vi "SpectrumAnalyzer.vi"() -> ()   [LabVIEW 2024]
uses:
  <vilib>/express/express analysis/Spectral/Block/exnSpectralBlock spectral measurements RMS poly.vi
  <vilib>/express/express analysis/Spectral/Block/exnSpectralBlock spectral measurements RMS WFM.vi
  <vilib>/express/express analysis/Spectral/XNode/ExpressSpectralMeasurementsBlockNode.xnode
  <vilib>/express/express analysis/Spectral/Block/exnSpectralBlock spectral measurements RMS DDT.vi
  <vilib>/Waveform/WDTOps.llb/WDT Waveform to XY Pairs DBL.vi
panel:
  out "Mic Wave 2":dynamicdata(graph) caption="Sine"
  out "mic+waves FFT":cluster{"f0":dbl, "df":dbl, "magnitude":dbl[]}(graph)
  out "Mic and waves SUM":waveform(dbl)(graph)
  in  "stop 2":bool
  in  "Simulate Waves Button":bool
  in  "Play Sound Button":bool
  out "Square Wave":dbl[](graph)
  out "Sine Wave":dbl[](graph)
  in  "Sin Coeffs":cluster{"freq":dbl, "Amp":dbl, "Phase":dbl}={"freq"=100.0, "Amp"=10.0, "Phase"=0.0}
  in  "Square Coeffs":cluster{"freq":dbl, "Amp":dbl, "Phase":dbl}={"freq"=100.0, "Amp"=10.0, "Phase"=0.0}
  in  "Sample Rate":dbl=44100.0
  in  "Duration":dbl=3.0
  in  "Signal Toggles":cluster{"Mic":bool, "Sin":bool, "Squ":bool}={"Mic"=TRUE, "Sin"=TRUE, "Squ"=TRUE}
  in  "Record Button":bool
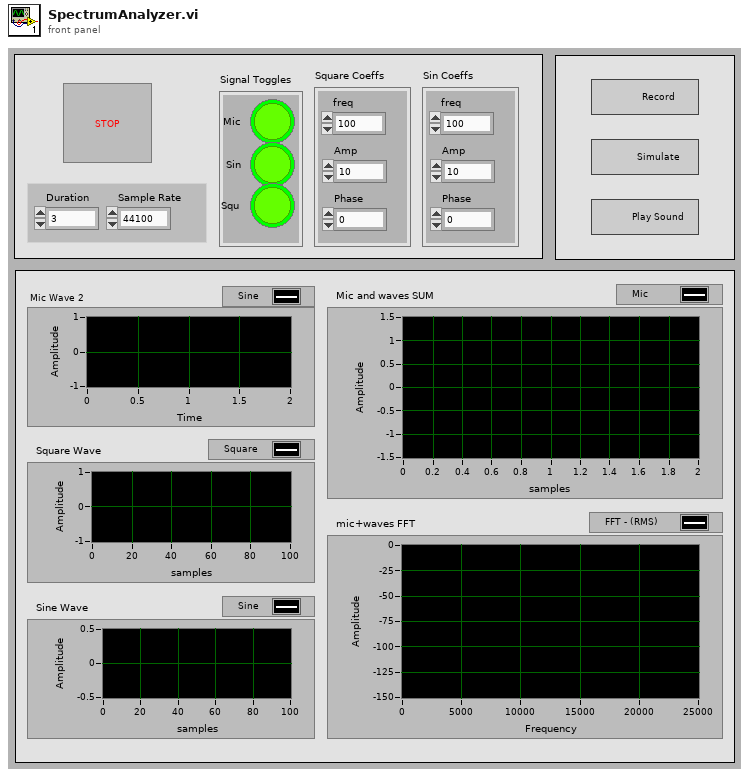
[diagram p1: front panel]
types:
  T1 = cluster{"averaging mode":u16, "weighting mode":u16, "number of averages":u32}
  T2 = cluster{"dB On (F)":bool, "unwrap phase (F)":bool, "convert to degree (F)":bool}
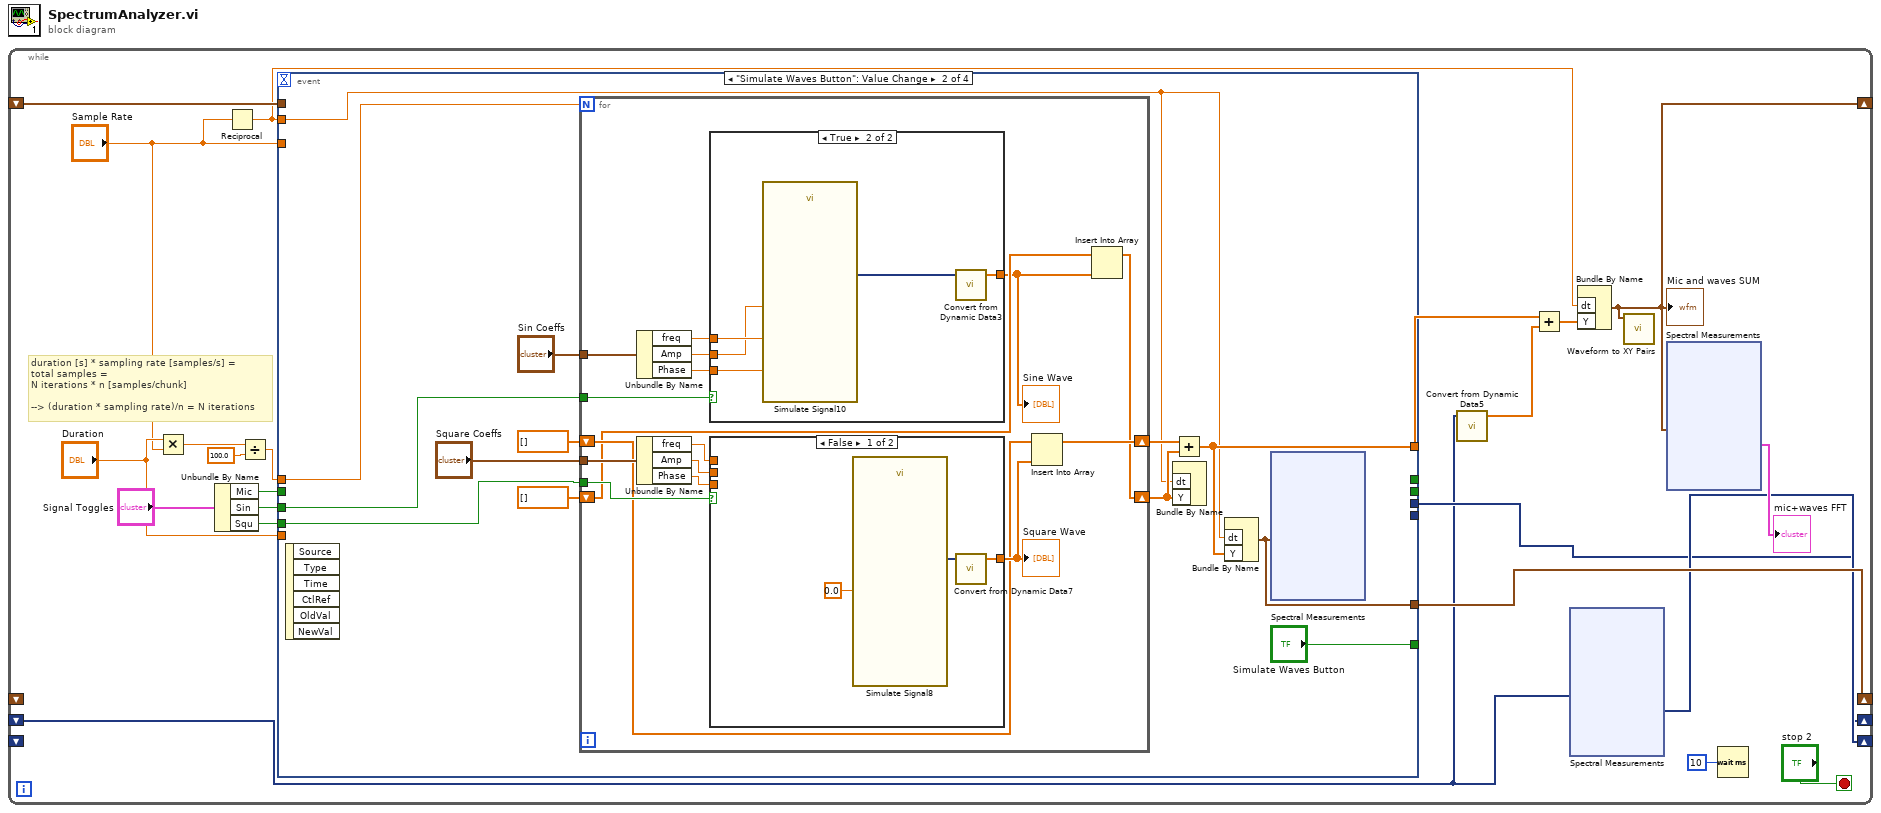
[diagram p0: block diagram]
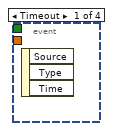
[diagram p2: hidden frame]
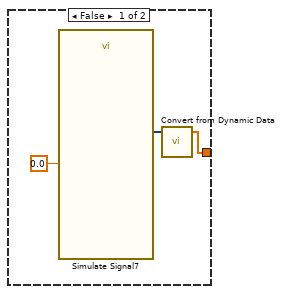
[diagram p3: hidden frame]
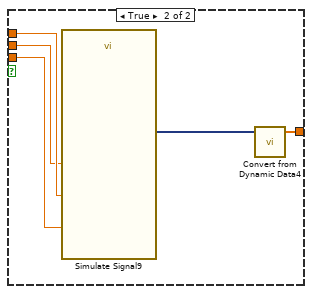
[diagram p4: hidden frame]
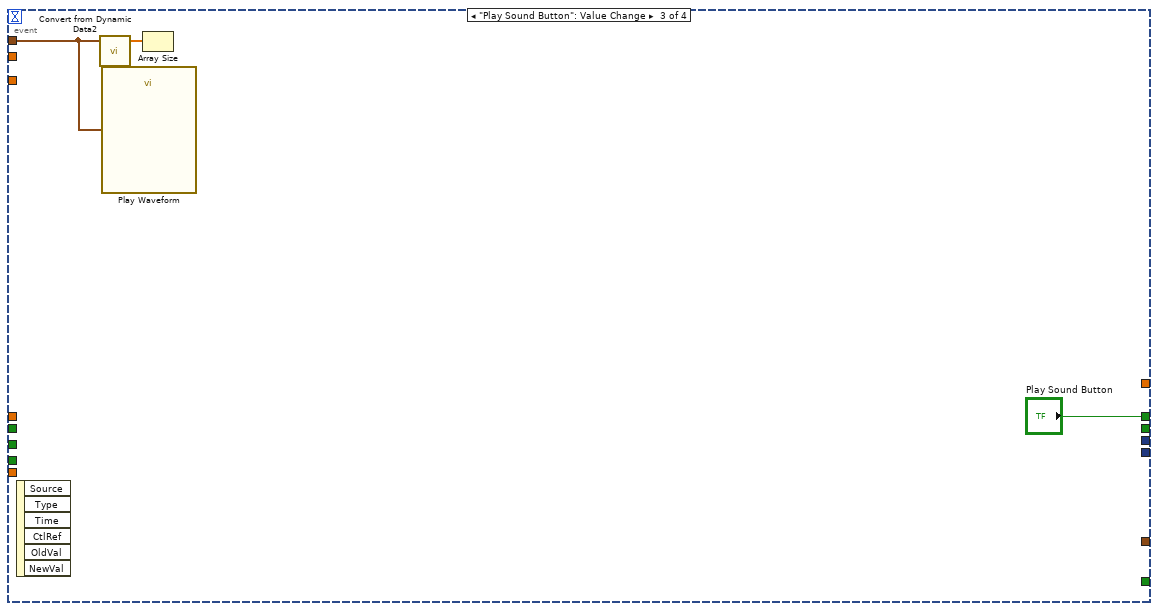
[diagram p5: hidden frame]
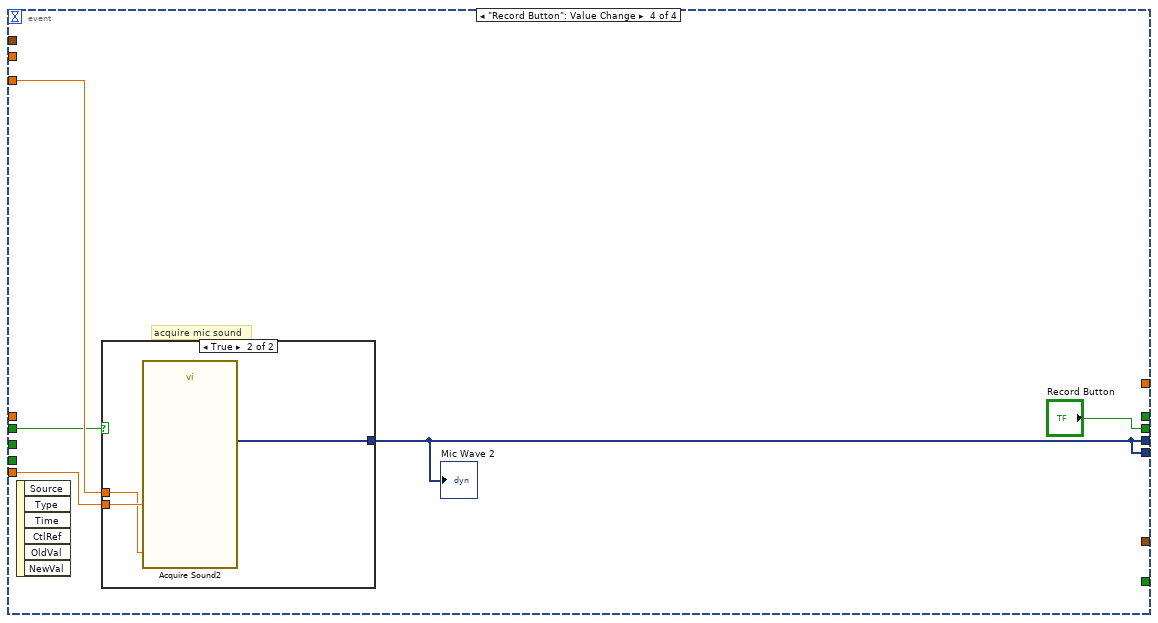
[diagram p6: hidden frame]
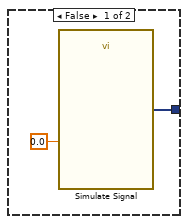
[diagram p7: hidden frame]
diagram:
  n1 = while {
    shift-right: [w8] -> _
    shift-left: _ -> [w15]
    shift-right: [w16] -> _
    shift-left: _ -> [_]
    shift-right: [w6] -> _
    shift-left: _ -> [w5]
    shift-right: [w7] -> _
    shift-left: _ -> [_]
    stop <- "stop 2" stop-if-true
    # "duration [s] * sampling rate [samples/s] =\ntotal samples =\nN iterations * n [samples/chunk] \n\n--> (duration * sampling rate)/n = N iterations"
    n2 = Multiply(x="Duration", y="Sample Rate") -> (x*y=w20:dbl)
    n3 = Unbundle By Name("Signal Toggles") -> ("Mic"=w3:bool, "Sin"=w2:bool, "Squ"=w1:bool)
    n4 = Reciprocal(x="Sample Rate") -> (1/x=w10:dbl)
    n5 = Divide(x=w20, y=100.0) -> (x/y=w18:dbl)
    n6 = event shown="[1] \"Simulate Waves Button\": Value Change" {
      selector: _ -> [_ _ _ _]
      dyn-events: _ -> [_ _ _ _]
      timeout: _ -> [_ _ _ _]
      tunnel: "Duration" -> [_ _ _ w105]
      tunnel: "Sample Rate" -> [_ _ _ w104]
      tunnel: w3 -> [_ _ _ w103]
      tunnel: w2 -> [_ w53 _ _]
      tunnel: w1 -> [_ w52 _ _]
      tunnel: w18 -> [_ w51 _ _]
      tunnel: [_ w50 _ _] -> w16
      tunnel: w15 -> [_ _ w98 _]
      tunnel: w10 -> [_ w43 _ _]
      tunnel: [_ _ _ w101] -> w6
      tunnel: [_ _ "Play Sound Button" _] -> _
      tunnel: [_ "Simulate Waves Button" _ _] -> _
      tunnel: [_ _ _ "Record Button"] -> _
      tunnel: [_ w44 _ _] -> w13
      tunnel: [_ _ _ w101] -> _
      event Timeout {
        n7 = event-data() -> ()  [unwired: 1 in, 3 out]
      }
      event "Simulate Waves Button": Value Change {
        n8 = event-data() -> ()  [unwired: 1 in, 6 out]
        n9 = for {
          N: w51 -> [_]
          tunnel: "Square Coeffs" -> [w81]
          tunnel: "Sin Coeffs" -> [w74]
          tunnel: w53 -> [w73]
          tunnel: w52 -> [w72]
          shift-right: [w70] -> w48
          shift-left: dbl[] [] -> [w69]
          shift-right: [w68] -> w47
          shift-left: dbl[] [] -> [w67]
          n10 = Unbundle By Name(w74) -> ("freq"=w77:dbl, "Amp"=w76:dbl, "Phase"=w75:dbl)
          n11 = Unbundle By Name(w81) -> ("freq"=w80:dbl, "Amp"=w79:dbl, "Phase"=w78:dbl)
          n12 = case shown="True" w73 {
            tunnel: [w82 w85] -> w66
            tunnel: w77 -> [_ w89]
            tunnel: w76 -> [_ w88]
            tunnel: w75 -> [_ w87]
            frame False {
              n13 = call "Simulate Signal7"("Amplitude"=0.0) -> ("Square"=w83:dynamicdata)  [unwired: 13 in, 1 out]
              n14 = call "Convert from Dynamic Data"("Dynamic Data Type"=w83) -> ("Array"=w82:dbl[])  [unwired: 3 in]
            }
            frame True {
              n15 = call "Simulate Signal10"("Frequency"=w89, "Amplitude"=w88, "Phase"=w87) -> ("Sine"=w86:dynamicdata)  [unwired: 11 in, 1 out]
              n16 = call "Convert from Dynamic Data3"("Dynamic Data Type"=w86) -> ("Array"=w85:dbl[])  [unwired: 3 in]
            }
          }
          "Sine Wave" <- w66
          n17 = case shown="False" w72 {
            tunnel: [w90 w93] -> w71
            tunnel: w80 -> [_ w97]
            tunnel: w79 -> [_ w96]
            tunnel: w78 -> [_ w95]
            frame False {
              n18 = call "Simulate Signal8"("Amplitude"=0.0) -> ("Square"=w91:dynamicdata)  [unwired: 13 in, 1 out]
              n19 = call "Convert from Dynamic Data7"("Dynamic Data Type"=w91) -> ("Array"=w90:dbl[])  [unwired: 3 in]
            }
            frame True {
              n20 = call "Simulate Signal9"("Frequency"=w97, "Amplitude"=w96, "Phase"=w95) -> ("Square"=w94:dynamicdata)  [unwired: 11 in, 1 out]
              n21 = call "Convert from Dynamic Data4"("Dynamic Data Type"=w94) -> ("Array"=w93:dbl[])  [unwired: 3 in]
            }
          }
          "Square Wave" <- w71
          n22 = Insert Into Array(array=w69, new element=w71) -> (w70:dbl[])  [unwired: 1 in]
          n23 = Insert Into Array(array=w67, new element=w66) -> (w68:dbl[])  [unwired: 1 in]
        }
        n24 = Bundle By Name("dt"=w43, "Y"=w47) -> ()  [unwired: 1 in, 1 out]
        n25 = Add(x=w48, y=w47) -> (x+y=w44:dbl[])
        n26 = Bundle By Name("dt"=w43, "Y"=w44) -> (w50:waveform(dbl))  [unwired: 1 in]
        n27 = xnode "Spectral Measurements"("Signals"=w50) -> ()  [unwired: 1 in, 3 out]
      }
      event "Play Sound Button": Value Change {
        n28 = event-data() -> ()  [unwired: 1 in, 6 out]
        n29 = call "Convert from Dynamic Data2"("Dynamic Data Type"=w98) -> ("Array"=w99:dbl[])  [unwired: 3 in]
        n30 = call "Play Waveform"("Data"=w98) -> ()  [unwired: 18 in, 1 out]
        n31 = Array Size(array=w99) -> ()  [unwired: 1 out]
      }
      event "Record Button": Value Change {
        # "acquire mic sound"
        n32 = event-data() -> ()  [unwired: 1 in, 6 out]
        n33 = case shown="True" w103 {
          tunnel: w105 -> [_ w110]
          tunnel: w104 -> [_ w109]
          tunnel: [w107 w108] -> w101
          frame False {
            n34 = call "Simulate Signal"("Amplitude"=0.0) -> ("Sine"=w107:dynamicdata)  [unwired: 13 in, 1 out]
          }
          frame True {
            n35 = call "Acquire Sound2"("Duration (s)"=w110, "Sample rate (Hz)"=w109) -> ("Data"=w108:dynamicdata)  [unwired: 16 in, 1 out]
          }
        }
        "Mic Wave 2" <- w101
      }
    }
    n36 = call "Convert from Dynamic Data5"("Dynamic Data Type"=w5) -> ("Array"=w12:dbl[])  [unwired: 3 in]
    n37 = Add(x=w13, y=w12) -> (x+y=w11:dbl[])
    n38 = xnode "Spectral Measurements"("Signals"=w5) -> ("FFT - (RMS)"=w7:dynamicdata)  [unwired: 1 in, 2 out]
    n39 = Bundle By Name("dt"=w10, "Y"=w11) -> (w8:waveform(dbl))  [unwired: 1 in]
    "Mic and waves SUM" <- w8
    n40 = call-poly <vilib>:"Waveform to XY Pairs.vi"("waveform in"=w8) -> ()  [unwired: 8 in, 3 out]
    n41 = xnode "Spectral Measurements"("Signals"=w8) -> ("FFT - (RMS)"=→"mic+waves FFT":cluster{"f0":dbl, "df":dbl, "magnitude":dbl[]})  [unwired: 1 in, 2 out]
    n42 = Wait (ms)(milliseconds to wait=u32 10) -> ()  [unwired: 1 out]
  }
